vi "reset.vi"(8 "error in (no error)":errorcluster, 9 "Monochromator in":refnum<class "Monochromator.lvclass">, 11 "ReadySate in":refnum<class "ReadySate.lvclass">) -> (0 "error out":errorcluster, 1 "Monochromator out":refnum<class "Monochromator.lvclass">, 3 "ReadySate out":refnum<class "ReadySate.lvclass">)   [LabVIEW 2016, in "ReadySate.lvclass"]
uses:
  ReadySate.lvclass
  Monochromator/Monochromator.lvclass
  Typedefs/AckType.ctl
  Typedefs/SWStatus.ctl
  Monochromator/Monochromator.lvclass/Monochromator.ctl
panel:
  in  "Force Init":bool
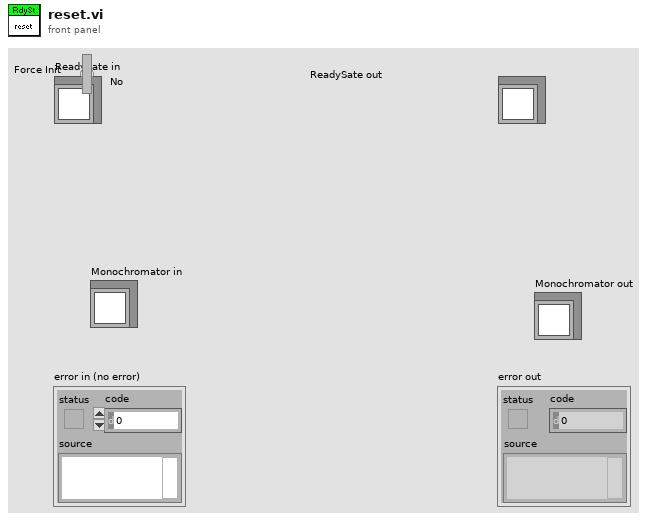
[diagram p1: front panel]
types:
  T1 = typedef "SWStatus.ctl" = enum16{"OfflineState", "ReadyState", "SettingUpState", "FaultState"}
  T2 = typedef "AckType.ctl" = enum16{"OK", "OutOfRange", "Unknown", "Busy", "Rejected"}
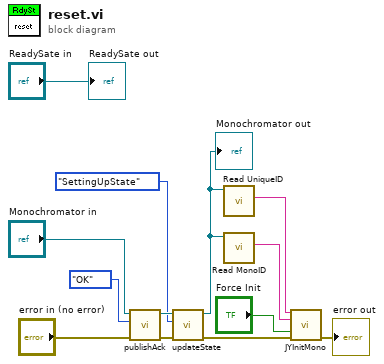
[diagram p0: block diagram]
diagram:
  n1 = call "publishAck.vi"("error in (no error)"="error in (no error)", "Ack"=AckType."OK" ("AckType"), "Monochromator in"="Monochromator in") -> ("error out"=w8:errorcluster, "Monochromator out"=w9:refnum<class "Monochromator.lvclass">)  [unwired: 7 in]
  n2 = call "updateState.vi"("error in (no error)"=w8, "SWStatus"=SWStatus."SettingUpState", "Monochromator in"=w9) -> ("error out"=w7:errorcluster, "Monochromator out"=w1:refnum<class "Monochromator.lvclass">)  [unwired: 7 in]
  "Monochromator out" <- w1
  n3 = call "Read UniqueID.vi"("Monochromator in"=w1) -> ("UniqueID"=w13:string)  [unwired: 8 in, 2 out]
  n4 = call "Read MonoID.vi"("Monochromator in"=w1) -> ("MonoID"=w12:string)  [unwired: 8 in, 2 out]
  n5 = call "JYInitMono.vi"("Unique ID"=w13, "Mono ID"=w12, "Force Init"="Force Init", "error in (no error)"=w7) -> ("error out"=→"error out":errorcluster)  [unwired: 7 in, 4 out]
  "ReadySate out" <- "ReadySate in"
